vi "Type Panel.vi"(11 "RelationPanel in":refnum<class "RelationPanel.lvclass">) -> ()   [LabVIEW 2020, in "Conditum-Tools.lvlib" / "RelationPanel.lvclass"]
uses:
  RelationPanel.lvclass
  C:/dev/lv20CE/lv-conditum-tools/Conditum-Tools/ColumnPanel/ColumnPanel.lvclass
  RelationPanel.lvclass/RelationPanel.ctl
  Conditum-Clone/Columns/Relation/Relation.lvclass
  Conditum-Clone/Columns/Relation/Relation.lvclass/Relation.ctl
  Available Entity.ctl
  ColumnPanel/ColumnPanel.lvclass
  Conditum-Tools.lvlib
panel:
  in  "Custom Reversed By?":bool
  in  "Related is Array":bool
  in  "Reversed By":string
  in  "This is Array":bool
  in  "Related To":string(combo)
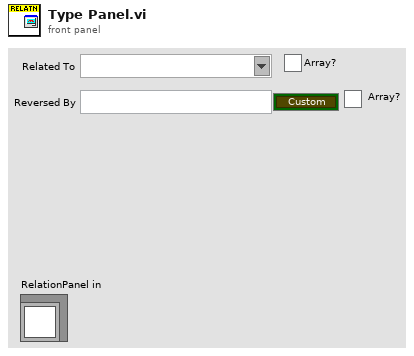
[diagram p1: front panel]
types:
  T1 = typedef "Conditum-Tools.lvlib/ColumnPanel.lvclass/Type Panel Event Reg.ctl" = refnum<event-registration>
  T2 = typedef "Conditum-Tools.lvlib/Available Entity.ctl" = cluster{"Class":string, "Name":string}
  T3 = enum8{"Enabled", "Disabled", "Disabled and Grayed Out"}
  T4 = typedef "Conditu2.lvlib/Relation Info.ctl" = cluster{"Mapping":T5, "Related To":string, "Reversed By":string, "Related Class":string}
  T5 = typedef "Conditu2.lvlib/Relation Mapping.ctl" = enum16{"OneToOne", "OneToMany", "ManyToOne", "ManyToMany"}
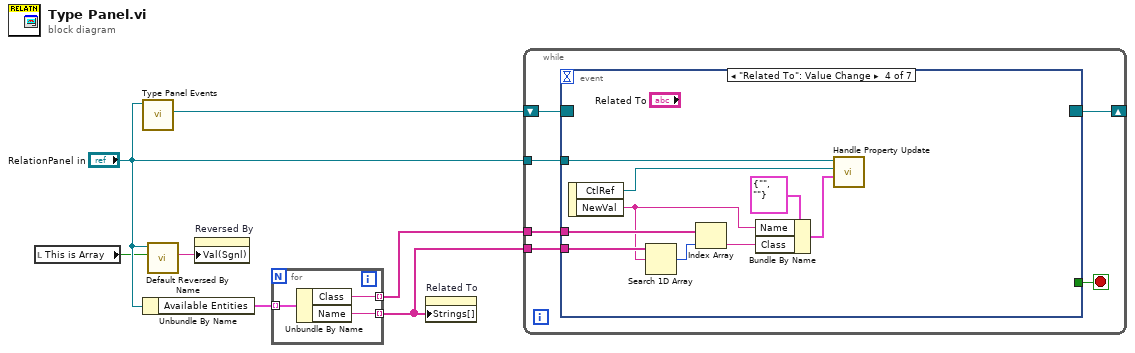
[diagram p0: block diagram]
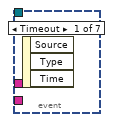
[diagram p2: hidden frame]
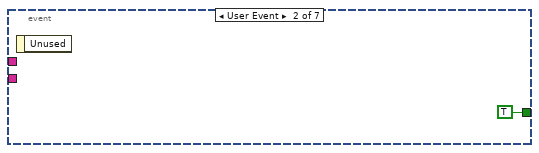
[diagram p3: hidden frame]
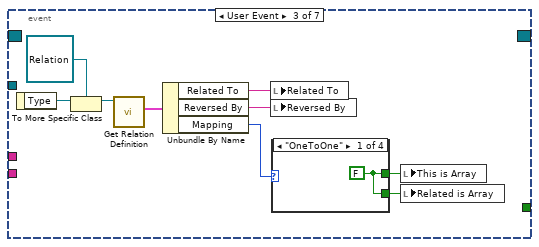
[diagram p4: hidden frame]
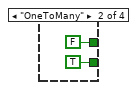
[diagram p5: hidden frame]
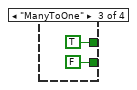
[diagram p6: hidden frame]
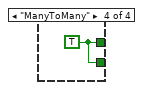
[diagram p7: hidden frame]
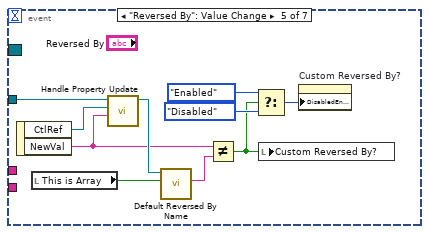
[diagram p8: hidden frame]
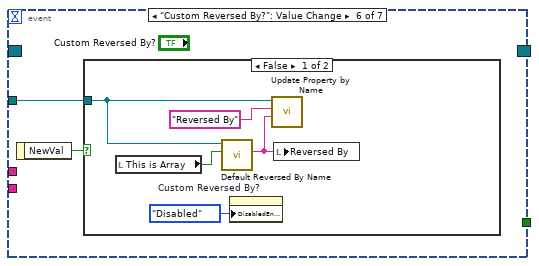
[diagram p9: hidden frame]
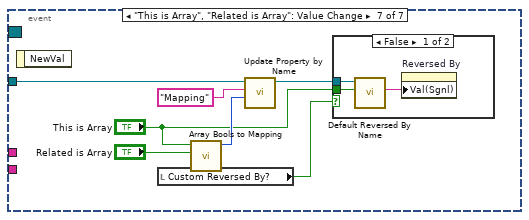
[diagram p11: hidden frame]
diagram:
  n1 = local read "This is Array"() -> (w4:bool)
  n2 = call "Type Panel Events.vi"("ColumnPanel"="RelationPanel in") -> ("Type Panel Event Reg"=w7:T1)  [unwired: 10 in]
  n3 = Unbundle By Name("RelationPanel in") -> ("Available Entities"=w3:T2[])
  n4 = call "Default Reversed By Name.vi"("This is Array?"=w4, "RelationPanel in"="RelationPanel in") -> ("Default Reversed By"=w5:string)  [unwired: 9 in]
  n5 = property on="Reversed By" class="Str"("Val(Sgnl)"=w5) -> ()  [unwired: 2 in, 2 out]
  n6 = for {
    tunnel: w3 -> [w10] mode=indexing
    tunnel: [w9] -> w2 mode=indexing
    tunnel: [w8] -> w1 mode=indexing
    n7 = Unbundle By Name(w10) -> ("Class"=w9:string, "Name"=w8:string)
  }
  n8 = property on="Related To" class="CmbBox"("Strings[]"=w1) -> ()  [unwired: 2 in, 2 out]
  n9 = while {
    tunnel: "RelationPanel in" -> [w15]
    shift-right: [w13] -> _
    shift-left: w7 -> [w14]
    tunnel: w2 -> [w12]
    tunnel: w1 -> [w11]
    stop <- w16 stop-if-true
    n10 = event shown="[3] \"Related To\": Value Change" {
      selector: w14 -> [_ _ _ _ _ _ _]
      dyn-events: [_ _ _ _ _ _ _] -> w13
      timeout: _ -> [_ _ _ _ _ _ _]
      tunnel: [_ TRUE _ _ _ _ _] -> w16
      tunnel: w15 -> [_ _ _ w41 w51 w52 w65]
      tunnel: w12 -> [_ _ _ w38 _ _ _]
      tunnel: w11 -> [_ _ _ w39 _ _ _]
      event Timeout {
        n11 = event-data() -> ()  [unwired: 1 in, 3 out]
      }
      event User Event {
        n12 = event-data() -> ()  [unwired: 1 in, 1 out]
      }
      event User Event {
        n13 = event-data() -> ("Type"=w26:refnum<class "Type.lvclass">)  [unwired: 1 in]
        n14 = To More Specific Class(target class=refnum<class "Relation.lvclass"> refnum ("Boolean"), reference=w26) -> (specific class reference=w19:refnum<class "Relation.lvclass">)  [unwired: 1 in, 1 out]
        n15 = call "Get Relation Definition.vi"("Relation in"=w19) -> ("Relation"=w18:T4)  [unwired: 10 in]
        n16 = Unbundle By Name(w18) -> ("Related To"=w24:string, "Reversed By"=w23:string, "Mapping"=w22:T5)
        n17 = local write "Related To"(w24) -> ()
        n18 = local write "Reversed By"(w23) -> ()
        n19 = case shown="\"OneToOne\"" w22 {
          tunnel: [w27 FALSE TRUE w32] -> w21
          tunnel: [w27 TRUE FALSE w32] -> w20
          frame "OneToOne" {
            w27 = FALSE
          }
          frame "OneToMany" {
          }
          frame "ManyToOne" {
          }
          frame "ManyToMany" {
            w32 = TRUE
          }
        }
        n20 = local write "This is Array"(w21) -> ()
        n21 = local write "Related is Array"(w20) -> ()
      }
      event "Related To": Value Change {
        n22 = event-data() -> ("CtlRef"=w40:refnum<vi>, "NewVal"=w34:string)  [unwired: 1 in]
        n23 = Search 1D Array(1D array=w39, element=w34) -> (index of element=w37:i32)  [unwired: 1 in]
        n24 = Index Array(array=w38, index=w37) -> (element=w35:string)
        n25 = Bundle By Name(cluster=T2 {"Class"="", "Name"=""} ("Available Entity"), "Name"=w34, "Class"=w35) -> (w33:T2)
        n26 = call "Handle Property Update.vi"("Value"=w33, "Control"=w40, "ColumnPanel in"=w41) -> ()  [unwired: 7 in, 2 out]
      }
      event "Reversed By": Value Change {
        n27 = event-data() -> ("CtlRef"=w50:refnum<vi>, "NewVal"=w47:string)  [unwired: 1 in]
        n28 = local read "This is Array"() -> (w49:bool)
        n29 = call "Handle Property Update.vi"("Value"=w47, "Control"=w50, "ColumnPanel in"=w51) -> ("ColumnPanel out"=w48:refnum<class "RelationPanel.lvclass">)  [unwired: 7 in, 1 out]
        n30 = call "Default Reversed By Name.vi"("This is Array?"=w49, "RelationPanel in"=w48) -> ("Default Reversed By"=w46:string)  [unwired: 9 in]
        n31 = Not Equal?(x=w47, y=w46) -> (x != y?=w43:bool)
        n32 = Select(t=T3."Enabled" ("Disabled"), s=w43, f=T3."Disabled" ("Disabled")) -> (s? t:f=w42:T3)
        n33 = local write "Custom Reversed By?"(w43) -> ()
        n34 = property on="Custom Reversed By?" class="Bool (strict)"("DisabledEnum"=w42) -> ()  [unwired: 2 in, 2 out]
      }
      event "Custom Reversed By?": Value Change {
        n35 = event-data() -> ("NewVal"=w53:bool)  [unwired: 1 in]
        n36 = case shown="False" w53 {
          tunnel: w52 -> [w56 _]
          frame False {
            n37 = local read "This is Array"() -> (w55:bool)
            n38 = call "Default Reversed By Name.vi"("This is Array?"=w55, "RelationPanel in"=w56) -> ("Default Reversed By"=w54:string)  [unwired: 9 in]
            n39 = property on="Custom Reversed By?" class="Bool (strict)"("DisabledEnum"=T3."Disabled" ("Disabled")) -> ()  [unwired: 2 in, 2 out]
            n40 = call "Update Property by Name.vi"("Value"=w54, "Name"="Reversed By", "ColumnPanel in"=w56) -> ()  [unwired: 7 in, 2 out]
            n41 = local write "Reversed By"(w54) -> ()
          }
          frame True {
          }
        }
      }
      event "This is Array", "Related is Array": Value Change {
        n42 = event-data() -> ()  [unwired: 1 in, 1 out]
        n43 = local read "Custom Reversed By?"() -> (w59:bool)
        n44 = call "Array Bools to Mapping.vi"("Related is Array"="Related is Array", "This is Array"="This is Array") -> ("Relation Mapping"=w62:T5)  [unwired: 9 in]
        n45 = call "Update Property by Name.vi"("Value"=w62, "Name"="Mapping", "ColumnPanel in"=w65) -> ("ColumnPanel out"=w61:refnum<class "RelationPanel.lvclass">)  [unwired: 7 in, 1 out]
        n46 = case shown="False" w59 {
          tunnel: w61 -> [w67 _]
          tunnel: "This is Array" -> [w66 _]
          frame False {
            n47 = call "Default Reversed By Name.vi"("This is Array?"=w66, "RelationPanel in"=w67) -> ("Default Reversed By"=w68:string)  [unwired: 9 in]
            n48 = property on="Reversed By" class="Str"("Val(Sgnl)"=w68) -> ()  [unwired: 2 in, 2 out]
          }
          frame True {
          }
        }
      }
    }
  }
